vi "ULx Read (Analog 1D Wfm NChan 1Samp).vi"(0 "task in":refnum<k24>, 9 "timeout":dbl=10.0 format="%_4g", 11 "error in":errorcluster) -> (4 "task out":refnum<k24>, 6 "data":waveform(dbl)[](array[waveform]), 15 "error out":errorcluster)   [LabVIEW 2020]
doc: "Reads a waveform that contains a single sample from each channel in a task that contains one or more analog input channels."
uses:
  C:/Users/William/Documents/LV 2020 builds/LeaktestDAQ/Source-v33/ULx_LV.dll
  ULx_LV.dll
panel:
  # "channel"
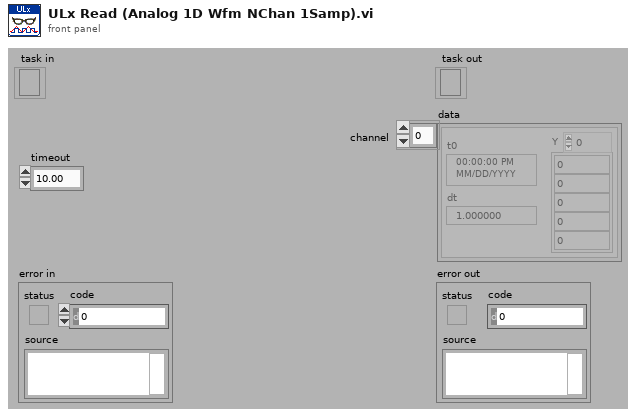
[diagram p1: front panel]
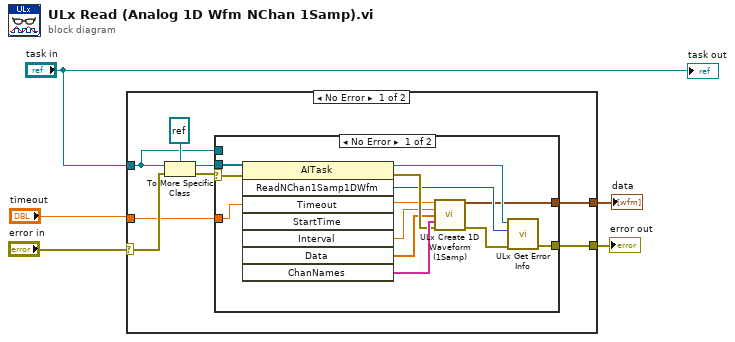
[diagram p0: block diagram]
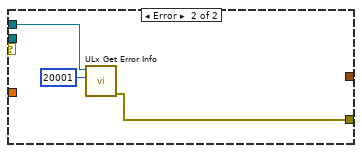
[diagram p2: hidden frame]
diagram:
  n1 = case shown="No Error" "error in" {
    selector: "error in" -> [w13 w30]
    tunnel: "task in" -> [w6 _]
    tunnel: "timeout" -> [w9 _]
    tunnel: [w8 w30] -> w3
    tunnel: [w7 _] -> w1
    frame No Error {
      n2 = To More Specific Class(target class=refnum<k24> refnum, reference=w6, error in=w13) -> (specific class reference=w10:refnum<k24>, error out=w11:errorcluster)
      n3 = case shown="No Error" w11 {
        selector: w11 -> [w25 _]
        tunnel: w10 -> [w26 _]
        tunnel: w9 -> [w22 _]
        tunnel: [w23 w28] -> w8
        tunnel: [w14 _] -> w7
        tunnel: w6 -> [_ w29]
        frame No Error {
          n4 = invoke class="AITask" method="ReadNChan1Samp1DWfm"(reference=w26, error in=w25, "Timeout"=w22) -> (reference out=w24:refnum<k24>, error out=w20:errorcluster, "ReadNChan1Samp1DWfm"=w15:i32, "StartTime"=w18:dbl, "Interval"=w17:dbl, "Data"=w16:dbl[], "ChanNames"=w21:string[])  [unwired: 5 in, 1 out]
          n5 = call "ULx Create 1D Waveform (1Samp).vi"("t0"=w18, "dt"=w17, "data Array"=w16, "channelName Array"=w21, "error in"=w20) -> ("data"=w14:waveform(dbl)[], "error out"=w19:errorcluster)  [unwired: 9 in]
          n6 = call "ULx Get Error Info.vi"("error in"=w19, "ErrorCode"=w15, "task in"=w24) -> ("error out"=w23:errorcluster)  [unwired: 8 in]
        }
        frame Error {
          n7 = call "ULx Get Error Info.vi"("ErrorCode"=20001, "task in"=w29) -> ("error out"=w28:errorcluster)  [unwired: 9 in]
        }
      }
    }
    frame Error {
    }
  }
  "error out" <- w3
  "data" <- w1
  "task out" <- "task in"
